vi "write_log_data.vi"(8 "error in (no error)":errorcluster, 10 "Array in":string[](array[string]), 11 "appended path":path) -> (0 "error out":errorcluster, 1 "Boolean":bool, 2 "Array out":string[](array[string]), 3 "Path":path, 5 "data":string)   [LabVIEW 2019]
uses:
  <vilib>/Utility/file.llb/Write Delimited Spreadsheet (string).vi
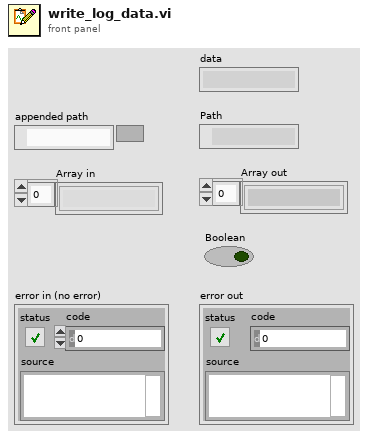
[diagram p1: front panel]
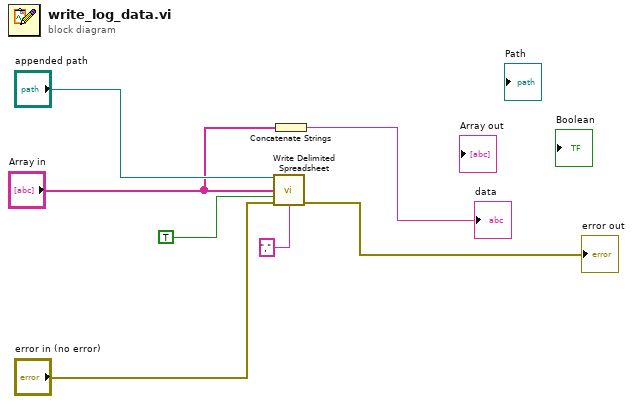
[diagram p0: block diagram]
diagram:
  n1 = call-poly <vilib>:"Write Delimited Spreadsheet.vi"("file path (dialog if empty)"="appended path", "1D data"="Array in", "append to file? (new file:F)"=TRUE, "error in (no error)"="error in (no error)", "delimiter (\\t)"="," ("delimiter (\\t)")) -> ("error out"=→"error out":errorcluster)  [unwired: 9 in, 1 out]
  n2 = Concatenate Strings("Array in") -> (→"data":string)
